vi "GetCodeLength.vi"(10 "code in":string, 11 "data in":string) -> (2 "code":string, 3 "length":i32, 5 "pass?":bool)   [LabVIEW 2018]
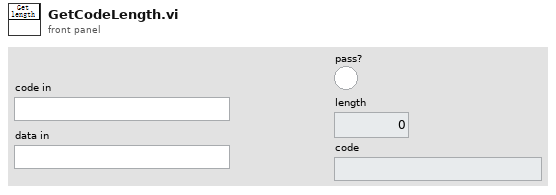
[diagram p1: front panel]
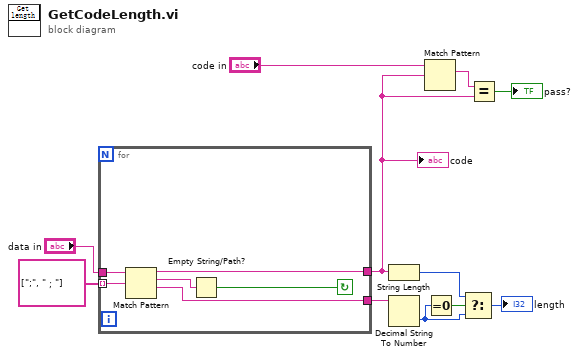
[diagram p0: block diagram]
diagram:
  n1 = for {
    tunnel: string[] [";", "；"] -> [w17] mode=indexing
    tunnel: [w15] -> w3
    tunnel: [w14] -> w9
    tunnel: "data in" -> [w13]
    stop <- w16 continue-if-true
    n2 = Match Pattern(string=w13, regular expression=w17) -> (before substring=w15:string, match substring=w12:string, after substring=w14:string)  [unwired: 1 in, 1 out]
    n3 = Empty String/Path?(string/path=w12) -> (empty?=w16:bool)
  }
  "code" <- w3
  n4 = String Length(string=w3) -> (length=w7:i32)
  n5 = Decimal String To Number(string=w9) -> (number=w6:i32)  [unwired: 2 in, 1 out]
  n6 = Match Pattern(string="code in", regular expression=w3) -> (match substring=w2:string)  [unwired: 1 in, 3 out]
  n7 = Equal To 0?(x=w6) -> (x = 0?=w8:bool)
  n8 = Select(t=w7, s=w8, f=w6) -> (s? t:f=→"length":i32)
  n9 = Equal?(x=w2, y=w3) -> (x = y?=→"pass?":bool)
